vi "Array Functions Part 3.vi"() -> ()   [LabVIEW 2020]
uses:
  0696d78d-884b-417d-84c4-2f530724673a.vi
  638bc39f-59d9-4a4a-b811-a616731044a2.vi
  d69dba08-f599-4cc4-83d0-42a01a8934d0.vi
  <vilib>/Comparison/Less/Less Functor/Less Functor.lvclass
  <vilib>/Comparison/Equal/Equal Functor/Equal Functor.lvclass
panel:
  out "reversed array":string[](array[string])
  out "index of element - not found":i32
  out "sorted array":string[](array[string])
  out "index of element":i32
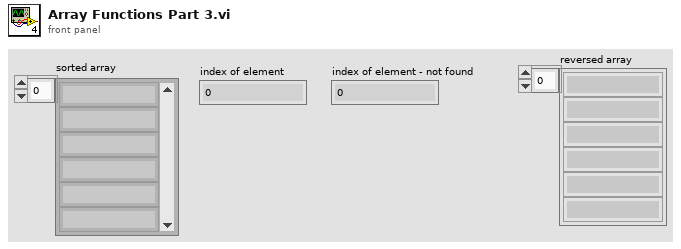
[diagram p1: front panel]
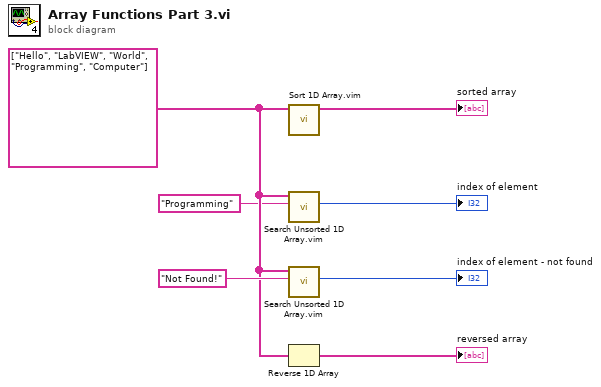
[diagram p0: block diagram]
diagram:
  w3 = string[] ["Hello", "LabVIEW", "World", "Programming", "Computer"]
  n1 = call "Sort 1D Array.vim"("unsorted array"=w3) -> ("sorted array"=→"sorted array":string[])  [unwired: 10 in]
  n2 = call "Search Unsorted 1D Array.vim"("element"="Programming" ("String"), "unsorted 1D array"=w3) -> ("index of element"=→"index of element":i32)  [unwired: 9 in]
  n3 = call "Search Unsorted 1D Array.vim"("element"="Not Found!" ("String"), "unsorted 1D array"=w3) -> ("index of element"=→"index of element - not found":i32)  [unwired: 9 in]
  n4 = Reverse 1D Array(array=w3) -> (reversed array=→"reversed array":string[])
